vi "Fine Tune Limbus Fit.vi"(7 "Grayscale Buffer 1":T1, 8 "error in":errorcluster, 9 "Results":T2={"Center X"=500, "Center Y"=500, "Radius X"=150, "Radius Y"=0, "Circle Match Score"=0, "Sclera Score"=0.0, "Circle Fit Strength"=0, "Circle Match Threshold"=0}, 10 "Treatment":T3, 11 "Green Plane":T1) -> (0 "error out":errorcluster, 1 "Results out":T2={"Center X"=500, "Center Y"=500, "Radius X"=150, "Radius Y"=0, "Circle Match Score"=0, "Sclera Score"=0.0, "Circle Fit Strength"=0, "Circle Match Threshold"=0})   [LabVIEW 2015]
uses:
  <vilib>/vision/Image Controls.llb/IMAQ Image.ctl
  controls/Treatment Parameters.ctl
  controls/Results.ctl
  <vilib>/vision/Measure.llb/Edge Options.ctl
  <vilib>/vision/Measure.llb/Edge Polarity.ctl
  <vilib>/vision/NI_Vision_Development_Module.lvlib
panel:
  in  "ROI Descriptor (Find Circular Edge 1)":T4={"Global Rectangle"=[557, 219, 946, 379], "Contours"=[{"ID"=enum."External", "Type"=7, "Coordinates"=[750, 155, 131, 223, 210635, 330382]}]} {"Contours"."Type" items=["No Selection", "Point", "Line", "Rectangle", "Oval", "Polygon", "Freehand Region", "Annulus", "Unused2", "Unused3", "Broken Line", "Freehand Line", "Rotated Rectangle"]}
  out "Image Out":T1(plugin-control)
  out "Fitted Circle (Find Circular Edge 1)":T5 {"Average SNR (dB)" format="%.2f"; "Average Strength" format="%.2f"; "Roundness (Real-World)" format="%.2f"; "Radius (Real-World)" format="%.2f"; "Center (Real-World)"."Y" format="%.2f"; "Center (Real-World)"."X" format="%.2f"; "Radius (Pixels)" format="%.2f"; "Center (Pixels)"."Y" format="%.2f"; "Center (Pixels)"."X" format="%.2f"}
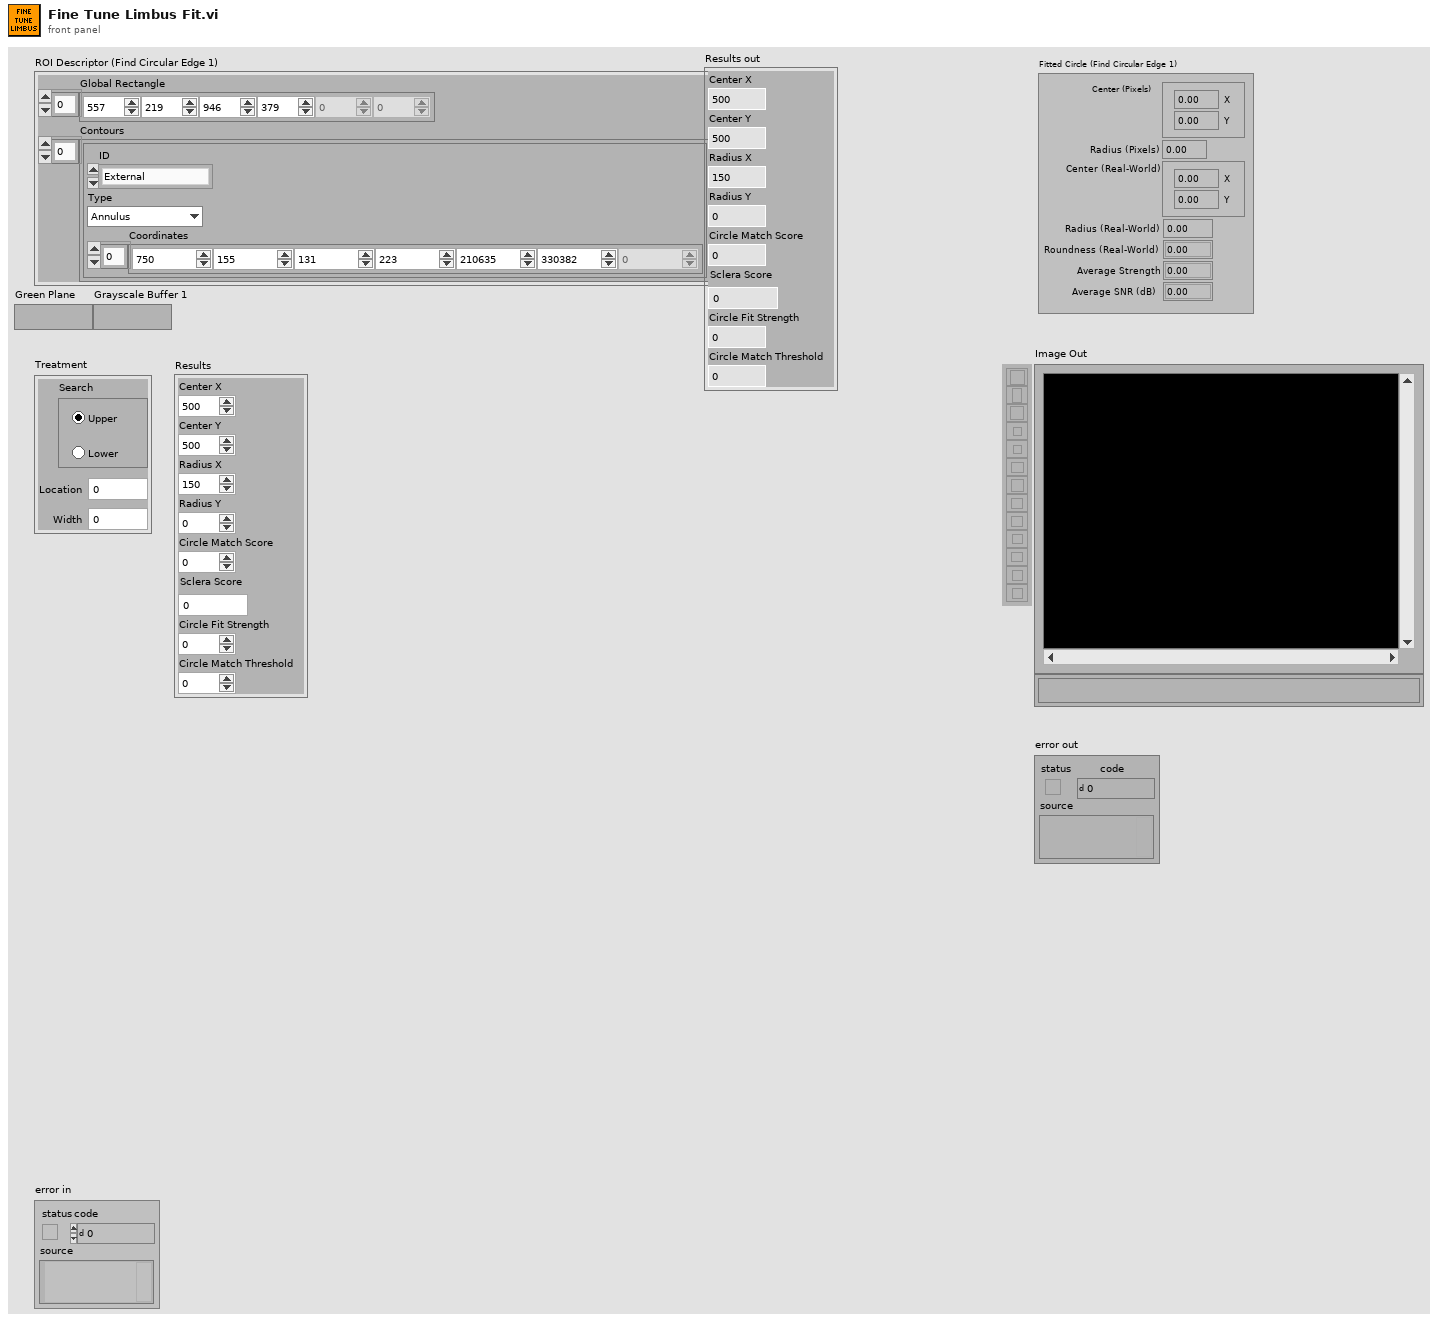
[diagram p1: front panel]
types:
  T1 = typedef "IMAQ Image.ctl" = refnum<image>
  T2 = typedef "Results.ctl" = cluster{"Center X":i32, "Center Y":i32, "Radius X":i32, "Radius Y":i32, "Circle Match Score":i32, "Sclera Score":dbl, "Circle Fit Strength":i32, "Circle Match Threshold":i32}
  T3 = typedef "Treatment Parameters.ctl" = cluster{"Location":dbl, "Width":dbl, "Search":enum32{"Upper", "Lower"}}
  T4 = cluster{"Global Rectangle":i32[], "Contours":cluster{"ID":enum32{"External", "Internal"}, "Type":u32, "Coordinates":i32[]}[]}
  T5 = cluster{"Center (Pixels)":cluster{"X":sgl, "Y":sgl}, "Radius (Pixels)":dbl, "Center (Real-World)":cluster{"X":sgl, "Y":sgl}, "Radius (Real-World)":dbl, "Roundness (Real-World)":dbl, "Average Strength":dbl, "Average SNR (dB)":dbl}
  T6 = typedef "IMAQ Circle" = cluster{"Center X":i32, "Center Y":i32, "Inner Radius":i32, "Outer Radius":i32, "Start Angle":dbl, "End Angle":dbl}
  T7 = cluster{"Process":enum16{"Get First Edge", "Get First + Last Edge", "Get All Edges", "Get Best Edge"}, "Step Size":i32, "Max Pixel Radius":i32}
  T8 = typedef "Edge Options.ctl" = cluster{"Edge Polarity":T9, "Kernel Size":u32, "Width":u32, "Minimum Edge Strength":sgl, "Interpolation Type":enum32{"Zero Order", "Bilinear", "Quadratic", "Cubic", "Bilinear Fixed"}, "Data Processing Method":enum32{"Average", "Median"}}
  T9 = typedef "Edge Polarity.ctl" = u32
  T10 = cluster{"Search  Direction":u32, "Edge Options":T8, "Show Search Area":bool, "Show Search Lines":bool, "Show Edges Found":bool, "Show Result":bool, "Search Area Color":u32, "Search Lines Color":u32, "Edge Locations Color":u32, "Result Color":u32, "Overlay Group Name":string}
  T11 = cluster{"histogram":u32[], "Minimal Value":sgl, "Maximal Value":sgl, "Starting Value":sgl, "Interval Width":sgl, "Mean Value":sgl, "Standard  Variation":sgl, "Area (pixels)":i32}
  T12 = typedef "Image Type" = u32
  T13 = typedef "ROI Descriptor" = cluster{"Global Rectangle":i32[], "Contours":cluster{"ID":enum32{"External", "Internal"}, "Type":u32, "Coordinates":i32[]}[]}
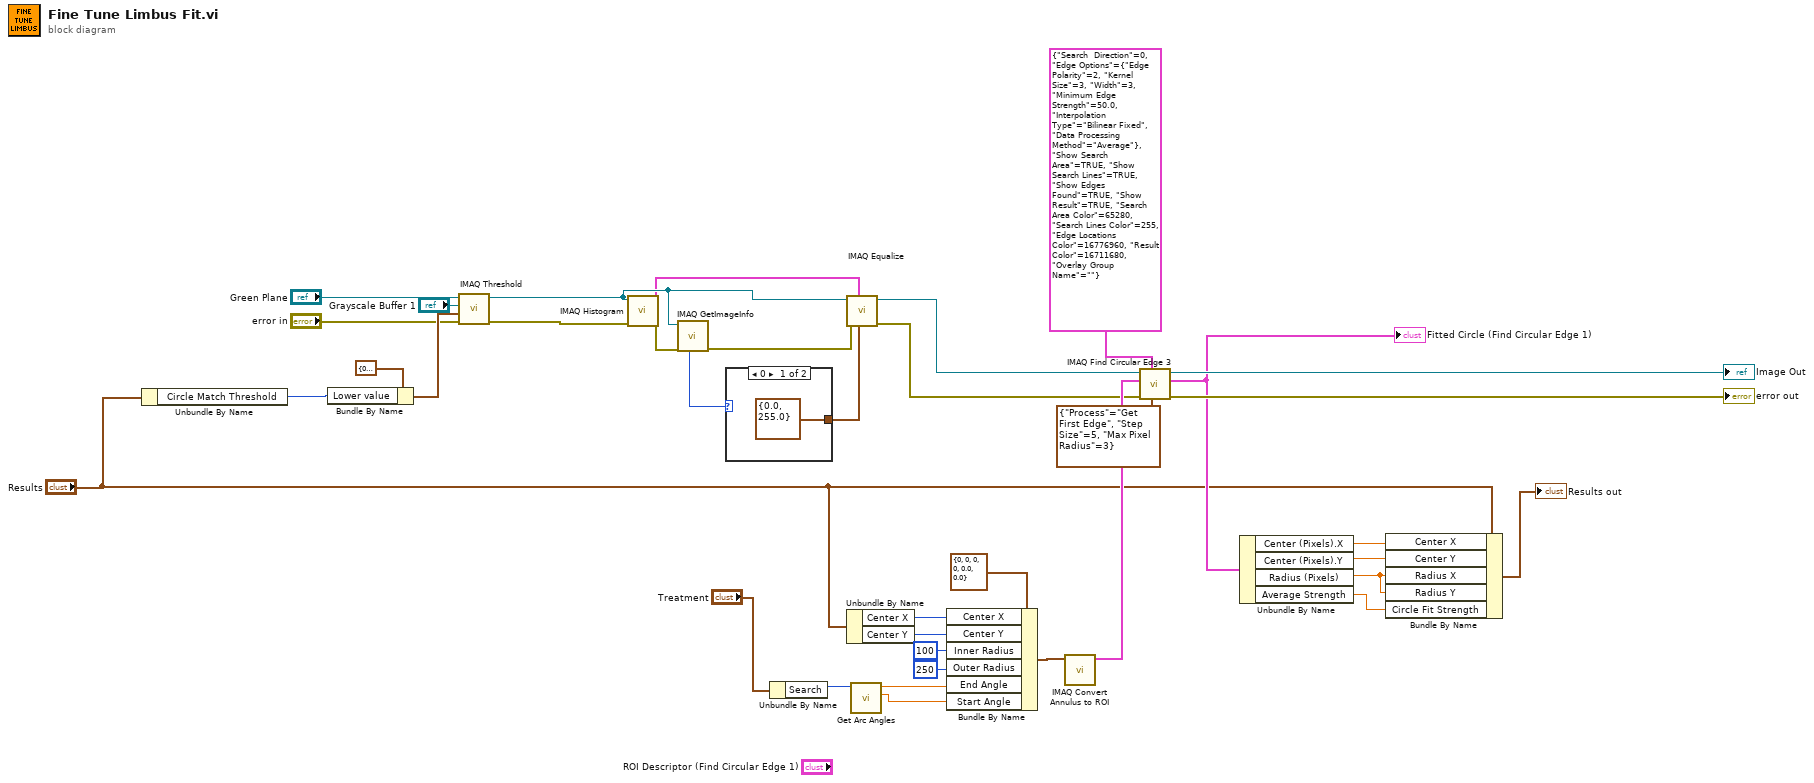
[diagram p0: block diagram]
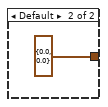
[diagram p2: hidden frame]
diagram:
  n1 = Unbundle By Name("Results") -> ("Circle Match Threshold"=w6:i32)
  n2 = Bundle By Name(cluster=cluster{"Lower value":sgl, "Upper value":sgl} {"Lower value"=0.0, "Upper value"=255.0} ("Range (Threshold 1)"), "Lower value"=w6) -> (w7:cluster{"Lower value":sgl, "Upper value":sgl})
  n3 = call "IMAQ Threshold"("error in (no error)"="error in", "Range"=w7, "Image Dst"="Grayscale Buffer 1", "Image Src"="Green Plane") -> ("error out"=w15:errorcluster, "Image Dst Out"=w14:T1)  [unwired: 2 in, 4 out]
  n4 = call "IMAQ Histogram"("error in (no error)"=w15, "Image"=w14) -> ("error out"=w11:errorcluster, "Histogram Report"=w13:T11)  [unwired: 3 in, 5 out]
  n5 = call "IMAQ GetImageInfo"("error in (no error)"=w11, "Image"=w14) -> ("error out"=w10:errorcluster, "Image Type"=w12:T12)  [unwired: 8 out]
  n6 = case shown="0" w12 {
    tunnel: [cluster{"Minimum":sgl, "Maximum":sgl} {"Minimum"=0.0, "Maximum"=255.0} ("Range") cluster{"Minimum":sgl, "Maximum":sgl} {"Minimum"=0.0, "Maximum"=0.0} ("Range")] -> w9
    frame 0 {
    }
    frame Default {
    }
  }
  n7 = Unbundle By Name("Treatment") -> ("Search"=w25:enum32{"Upper", "Lower"})
  n8 = call "IMAQ Equalize"("Range"=w9, "Histogram Report"=w13, "error in (no error)"=w10, "Image Src"=w14) -> ("error out"=w3:errorcluster, "Image Dst Out"=w5:T1)  [unwired: 2 in, 4 out]
  n9 = Unbundle By Name("Results") -> ("Center X"=w31:i32, "Center Y"=w30:i32)
  n10 = call "Get Arc Angles.vi"("Search Area"=w25) -> ("Start Angle (degrees)"=w23:dbl, "End Angle (degrees)"=w24:dbl)  [unwired: 9 in]
  n11 = Bundle By Name(cluster=T6 {"Center X"=0, "Center Y"=0, "Inner Radius"=0, "Outer Radius"=0, "Start Angle"=0.0, "End Angle"=0.0} ("Annulus"), "Center X"=w31, "Center Y"=w30, "Inner Radius"=100, "Outer Radius"=250, "End Angle"=w24, "Start Angle"=w23) -> (w32:T6)
  n12 = call "IMAQ Convert Annulus to ROI"("Annulus"=w32) -> ("ROI Descriptor"=w29:T13)  [unwired: 8 in, 1 out]
  n13 = call "IMAQ Find Circular Edge 3"("Circle Fit Options"=T7 {"Process"=enum."Get First Edge", "Step Size"=5, "Max Pixel Radius"=3} ("Circle Fit Options (Find Circular Edge 1)"), "Options"=T10 {"Search  Direction"=0, "Edge Options"={"Edge Polarity"=2, "Kernel Size"=3, "Width"=3, "Minimum Edge Strength"=50.0, "Interpolation Type"=enum."Bilinear Fixed", "Data Processing Method"=enum."Average"}, "Show Search Area"=TRUE, "Show Search Lines"=TRUE, "Show Edges Found"=TRUE, "Show Result"=TRUE, "Search Area Color"=65280, "Search Lines Color"=255, "Edge Locations Color"=16776960, "Result Color"=16711680, "Overlay Group Name"=""} ("Options (Find Circular Edge 1)"), "error in (no error)"=w3, "ROI Descriptor"=w29, "Image"=w5) -> ("error out"=→"error out":errorcluster, "Fitted Circle"=w22:T5, "Image Out"=→"Image Out":T1)  [unwired: 2 in, 2 out]
  "Fitted Circle (Find Circular Edge 1)" <- w22
  n14 = Unbundle By Name(w22) -> ("Center (Pixels).X"=w20:sgl, "Center (Pixels).Y"=w19:sgl, "Radius (Pixels)"=w18:dbl, "Average Strength"=w17:dbl)
  n15 = Bundle By Name(cluster="Results", "Center X"=w20, "Center Y"=w19, "Radius X"=w18, "Radius Y"=w18, "Circle Fit Strength"=w17) -> (→"Results out":T2)
